vi "Handle Command.vi"(8 "error in":errorcluster, 10 "CMD in":refnum<class "Change Speaker State CMD.lvclass">, 11 "Object In":refnum<class>) -> (0 "error out":errorcluster, 1 "Command Successful?":bool, 2 "CMD out":refnum<class "Change Speaker State CMD.lvclass">, 3 "Object Out":refnum<class>)   [LabVIEW 2017, in "gPAS Library.lvlib" / "Change Speaker State CMD.lvclass"]
doc: "This VI will contain the code used to actually execute the request. If the request is successful, this will be indicated by the boolean output <b>Command Successful?</b>. The boolean output can then be used by the <b>Command Reply</b> which sends a reply if the reply queue is valid."
uses:
  Change Speaker State CMD.lvclass
  C:/Program Files (x86)/National Instruments/LabVIEW 2017/vi.lib/MSR Consulting, LLC/General Reuse/PAS/Commands/Change Speaker State CMD/Change Speaker State CMD.lvclass
  nPAS.lvclass
  C:/Program Files (x86)/National Instruments/LabVIEW 2017/vi.lib/MSR Consulting, LLC/General Reuse/Instrument/Instrument.lvclass
  Global FPGA DO.ctl
  <vilib>/MSR Consulting, LLC/General Reuse/Instrument/Instrument.lvclass/Instrument.ctl
  nPAS.lvclass/nPAS.ctl
  <vilib>/MSR Consulting, LLC/General Reuse/PAS/Commands/Change Speaker State CMD/Change Speaker State CMD.lvclass/Change Speaker State CMD.ctl
  Change Laser Frequency Cmd/Change Laser Frequency CMD.lvclass
  C:/Program Files (x86)/National Instruments/LabVIEW 2017/vi.lib/MSR Consulting, LLC/General Reuse/Command/Command.lvclass
  Change Laser Frequency Cmd/Change Laser Frequency CMD.lvclass/Change Laser Frequency CMD.ctl
  Change Laser Frequency Cmd/Write f.vi
  Change Laser Frequency Cmd/Write Cell.vi
  <vilib>/MSR Consulting, LLC/General Reuse/PAS/Commands/Change Speaker State CMD/Read state.vi
  <vilib>/MSR Consulting, LLC/General Reuse/PAS/Commands/Change Speaker State CMD/Read cell.vi
  <vilib>/MSR Consulting, LLC/General Reuse/Instrument/Read ExtCom.vi
  <vilib>/MSR Consulting, LLC/General Reuse/Instrument/Read Log Session.vi
  Accessors/Read hFPGA.vi
  <vilib>/MSR Consulting, LLC/General Reuse/Instrument/Read CMD.vi
  <vilib>/Utility/error.llb/Error Cluster From Error Code.vi
  <vilib>/rvi/errors/niLvFpgaAdjustHostInterfaceError.vi
  Global DO.vi
  <vilib>/MSR Consulting, LLC/General Reuse/Session APIs/_Session Fwk/Session - Root.lvclass
  <vilib>/MSR Consulting, LLC/General Reuse/Command/Command.lvclass
  <vilib>/rvi/interface/nirviReadWriteControl/nirviReadWriteControl.xnode
  FPGA Ref.ctl
  FPGA Bitfiles/server_v1_2_1_4.lvbitx
  <vilib>/MSR Consulting, LLC/General Reuse/PAS/Commands/Change Speaker State CMD/Change Speaker State CMD.lvclass
  <vilib>/MSR Consulting, LLC/General Reuse/Session APIs/Session Log/System Log.lvclass
  Session/Raw FPGA/FPGA Session.lvclass
  NiFpgaLv.dll
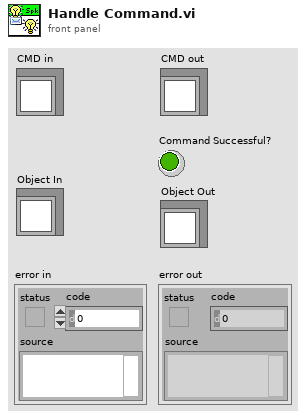
[diagram p1: front panel]
types:
  T1 = typedef "Global FPGA DO.ctl" = enum16{"pas_laser_relay_1", "pas_heater_1", "pas_heater_2", "pas_laser_relay_2", "pas_spk_enable_1", "pas_spk_enable_2", "hanbay_pos", "fan_enable", "crd_laser_enable", "crd_heater_enable", "vacuum_pump", "ac_spare", "uv_enable", "solenoid_1", "solenoid_2", "spare_dc_relay_1", "usb_hub_relay", "spare_dc_relay_2", "fp_aux_1", "fp_aux_2"}
  T2 = typedef "Session - Root.lvclass/Session Handle.ctl" = refnum<data-value>
  T3 = typedef "FPGA Ref.ctl" = refnum<k20>
  T4 = cluster{"tag":string, "section":string, "data":variant}
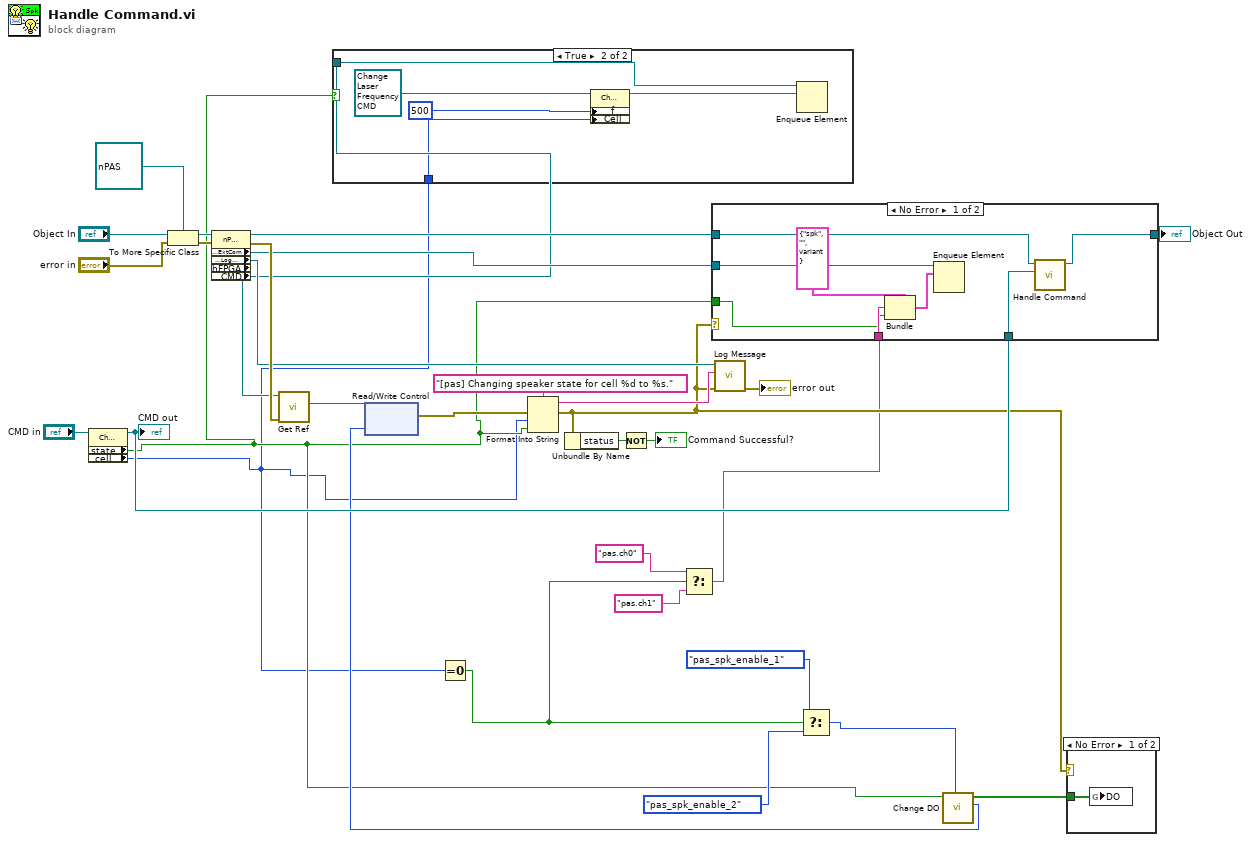
[diagram p0: block diagram]
diagram:
  n1 = property class="Change Speaker State CMD"(reference="CMD in") -> (reference out=w14:refnum<class "Change Speaker State CMD.lvclass">, "state"=w3:bool, "cell"=w1:u8)  [unwired: 1 in, 1 out]
  "CMD out" <- w14
  n2 = To More Specific Class(target class=refnum<class "nPAS.lvclass"> refnum ("nPAS"), reference="Object In", error in="error in") -> (specific class reference=w31:refnum<class "nPAS.lvclass">, error out=w28:errorcluster)
  n3 = property class="nPAS"(reference=w31, error in=w28) -> (reference out=w23:refnum<class "nPAS.lvclass">, error out=w27:errorcluster, "Accessors:ExtCom"=w19:refnum<queue>, "Accessors:Log Session"=w16:T2, "hFPGA"=w17:T2, "Accessors:CMD"=w2:refnum<queue>)
  n4 = call "Get Ref.vi"("error in"=w27, "Hanlde Out"=w17) -> ("FPGA Ref"=w26:T3)  [unwired: 7 in, 2 out]
  n5 = case shown="True" w3 {
    tunnel: w2 -> [_ w37]
    tunnel: w1 -> [_ w35]
    frame False {
    }
    frame True {
      n6 = property class="Change Laser Frequency CMD"(reference=refnum<class "Change Laser Frequency CMD.lvclass"> refnum ("gPAS Library.lvlib:Change Laser Frequency CMD"), "f"=u32 500, "Cell"=w35) -> (reference out=w36:refnum<class "Change Laser Frequency CMD.lvclass">)  [unwired: 1 in, 1 out]
      n7 = Enqueue Element(queue=w37, element=w36) -> ()  [unwired: 2 in, 3 out]
    }
  }
  n8 = Equal To 0?(x=w1) -> (x = 0?=w7:bool)
  n9 = Select(t="pas.ch0", s=w7, f="pas.ch1") -> (s? t:f=w4:string)
  n10 = Select(t=Global_FPGA_DO."pas_spk_enable_1" ("DO"), s=w7, f=Global_FPGA_DO."pas_spk_enable_2" ("DO")) -> (s? t:f=w10:T1)
  n11 = call "Change DO.vi"("DO"=w10, "val_in"=w3) -> ("DO Long Out"=w8:u32, "DO Out"=w13:bool[])  [unwired: 8 in]
  n12 = xnode "Read/Write Control"("FPGA VI Reference In"=w26, "DO"=w8) -> ("error out"=w25:errorcluster)  [unwired: 1 in, 1 out]
  n13 = Format Into String(format string="[pas] Changing speaker state for cell %d to %s.", error in=w25, w1, w3) -> (resulting string=w24:string, error out=w9:errorcluster)  [unwired: 1 in]
  n14 = Unbundle By Name(w9) -> ("status"=w22:bool)
  n15 = Not(x=w22) -> (.not. x?=→"Command Successful?":bool)
  n16 = case shown="No Error" w9 {
    tunnel: w23 -> [w43 w47]
    tunnel: w3 -> [w39 _]
    tunnel: w19 -> [w46 _]
    tunnel: [w42 w47] -> w15
    tunnel: w14 -> [w41 _]
    tunnel: w4 -> [w40 _]
    frame No Error {
      n17 = Bundle(cluster=T4 {"tag"="spk", "section"="", "data"=variant} ("element"), "section"=w40, "data"=w39) -> (w44:T4)  [unwired: 1 in]
      n18 = Enqueue Element(queue=w46, element=w44) -> ()  [unwired: 2 in, 3 out]
      n19 = call-parent "Handle Command.vi"("CMD in"=w41, "Object In"=w43) -> ("Object Out"=w42:refnum<class>)  [unwired: 6 in, 3 out]
    }
    frame Error {
    }
  }
  "Object Out" <- w15
  n20 = call <vilib>:"Log Message.vi"("error in"=w9, "MSG In"=w24, "session in"=w16) -> ("error out"=→"error out":errorcluster)  [unwired: 7 in, 1 out]
  n21 = case shown="No Error" w9 {
    tunnel: w13 -> [w48 _]
    frame No Error {
      n22 = global write "Global DO.vi" "DO"(w48) -> ()
    }
    frame Error {
    }
  }
